vi "toml_read_variant.vi"(7 "section":string[](array[string]), 8 "error in (no error)":errorcluster, 9 "default":variant, 10 "key":string[](array[string]), 11 "path in":path) -> (0 "error out":errorcluster, 1 "value":variant, 2 "exists?":bool, 3 "path out":path)   [LabVIEW 2017]
uses:
  <vilib>/Utility/Data Type/NI_Data Type.lvlib
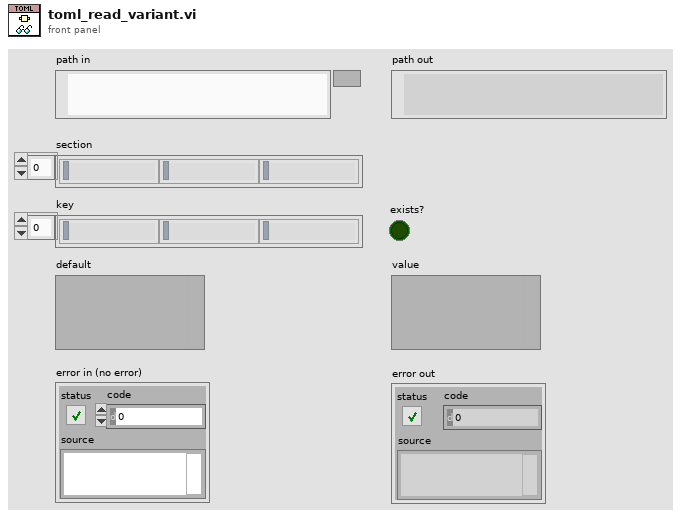
[diagram p1: front panel]
types:
  T1 = typedef "NI_Data Type.lvlib/Data Type.ctl" = enum8{"Invalid Type", "Void", "I8", "I16", "I32", "I64", "U8", "U16", "U32", "U64", "Single Float", "Double Float", "Extended Float", "Single Complex", "Double Complex", "Extended Complex", "Enum U8", "Enum U16", "Enum U32", "Enum U64", "Single Float With Unit", "Double Float With Unit", "Extended Float With Unit", "Single Complex with Unit", "Double Complex with Unit", "Extended Complex with Unit", "Boolean", "String", "Path", "Picture", "Tag", "Array", "Cluster", "Variant", "LV Variant", "Waveform", "Timestamp", "Digital Waveform", "Digital Data", "ExpressData", "Refnum", "External Data", "VI", "Poly VI", "LabVIEW Class Instance", "Fixed Point"}
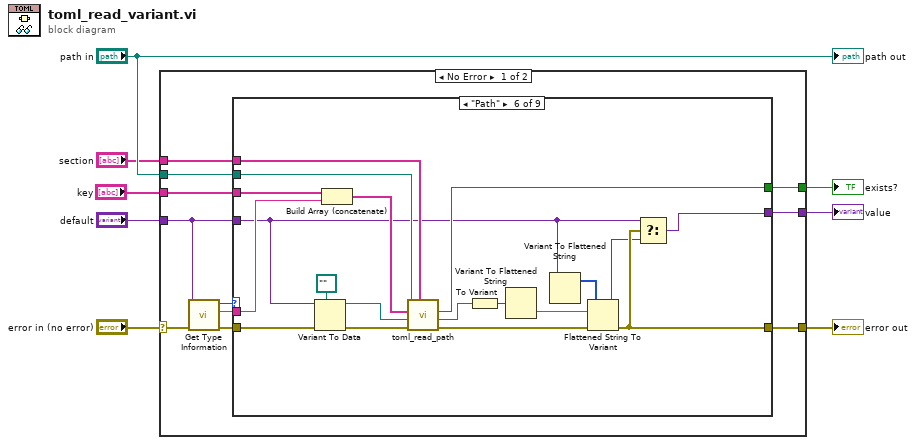
[diagram p0: block diagram]
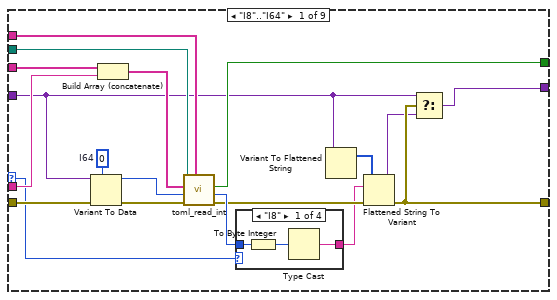
[diagram p2: hidden frame]
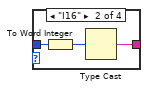
[diagram p3: hidden frame]
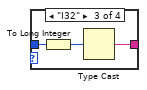
[diagram p4: hidden frame]
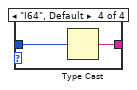
[diagram p5: hidden frame]
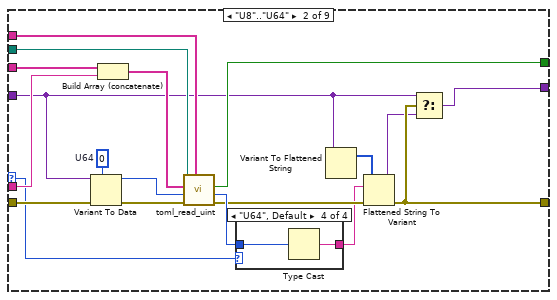
[diagram p6: hidden frame]
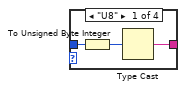
[diagram p7: hidden frame]
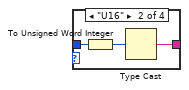
[diagram p8: hidden frame]
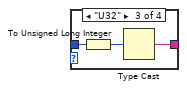
[diagram p9: hidden frame]
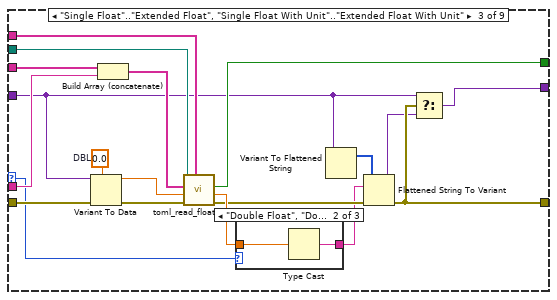
[diagram p10: hidden frame]
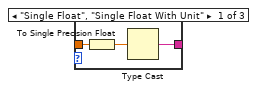
[diagram p11: hidden frame]
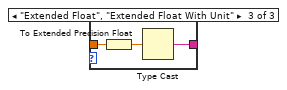
[diagram p12: hidden frame]
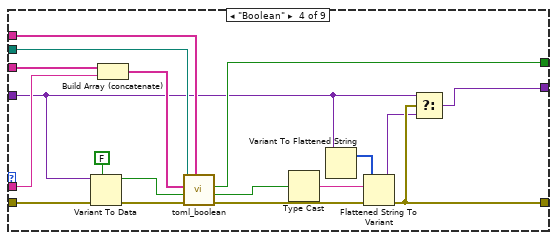
[diagram p13: hidden frame]
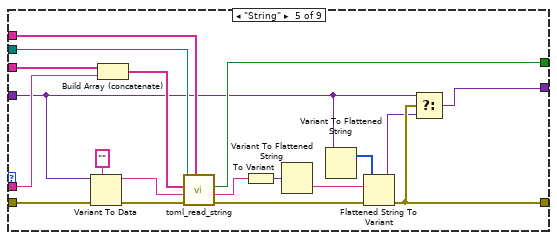
[diagram p14: hidden frame]
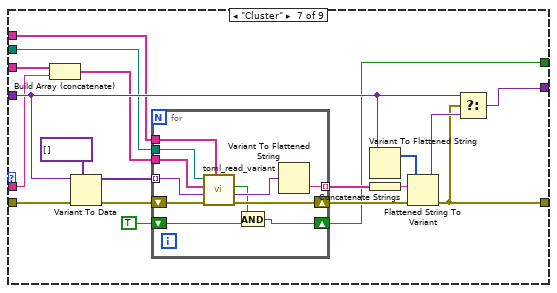
[diagram p15: hidden frame]
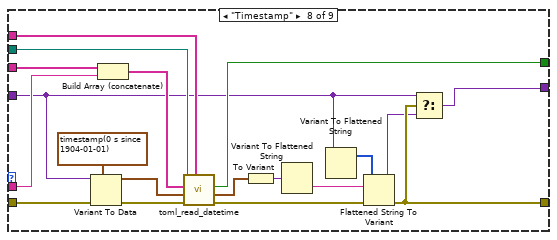
[diagram p16: hidden frame]
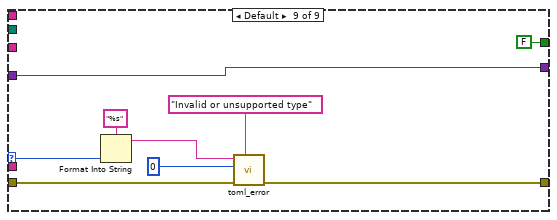
[diagram p17: hidden frame]
diagram:
  n1 = case shown="No Error" "error in (no error)" {
    selector: "error in (no error)" -> [w18 w222]
    tunnel: [w19 w222] -> w8
    tunnel: "default" -> [w16 w221]
    tunnel: [w14 w221] -> w5
    tunnel: "path in" -> [w13 _]
    tunnel: "section" -> [w11 _]
    tunnel: "key" -> [w10 _]
    tunnel: [w9 _] -> w1
    frame No Error {
      n2 = call <vilib>:"Get Type Information.vi"("error in (no error)"=w18, "Variant"=w16) -> ("error out"=w17:errorcluster, "Name"=w12:string, "Type"=w15:T1)  [unwired: 5 in, 2 out]
      n3 = case shown="\"Path\"" w15 {
        selector: w15 -> [w25 w55 w85 _ _ _ _ _ w216]
        tunnel: [w23 w53 w83 w110 w131 w150 w175 w199 w219] -> w19
        tunnel: w17 -> [w38 w68 w98 w124 w143 w162 w181 w211 w220]
        tunnel: w16 -> [w22 w52 w82 w109 w130 w149 w173 w198 w213]
        tunnel: [w20 w50 w80 w107 w128 w147 w174 w196 w213] -> w14
        tunnel: w13 -> [w37 w67 w97 w123 w142 w161 w169 w210 _]
        tunnel: w12 -> [w34 w64 w94 w120 w139 w158 w171 w207 _]
        tunnel: w11 -> [w36 w66 w96 w122 w141 w160 w168 w209 _]
        tunnel: w10 -> [w35 w65 w95 w121 w140 w159 w172 w208 _]
        tunnel: [w29 w59 w89 w115 w134 w153 w163 w202 FALSE ("exists?")] -> w9
        frame "I8".."I64" {
          w31 = i64 0  # I64
          n4 = Variant To Data(error in=w38, type=w31, Variant=w22) -> (data=w30:i64, error out=w32:errorcluster)
          n5 = Build Array (concatenate)(w35, w34) -> (w33:string[])
          n6 = call "toml_read_int.vi"("section"=w36, "error in (no error)"=w32, "default"=w30, "key"=w33, "path in"=w37) -> ("error out"=w27:errorcluster, "value"=w28:i64, "exists?"=w29:bool)  [unwired: 2 in, 2 out]
          n7 = case shown="\"I8\"" w25 {
            tunnel: [w39 w42 w45 w49] -> w24
            tunnel: w28 -> [w41 w44 w47 w48]
            frame "I8" {
              n8 = To Byte Integer(number=w41) -> (8bit integer=w40:i8)
              n9 = Type Cast(x=w40) -> (*(type *) &x=w39:string)  [unwired: 1 in]
            }
            frame "I16" {
              n10 = To Word Integer(number=w44) -> (16bit integer=w43:i16)
              n11 = Type Cast(x=w43) -> (*(type *) &x=w42:string)  [unwired: 1 in]
            }
            frame "I32" {
              n12 = To Long Integer(number=w47) -> (32bit integer=w46:i32)
              n13 = Type Cast(x=w46) -> (*(type *) &x=w45:string)  [unwired: 1 in]
            }
            frame "I64", Default {
              n14 = Type Cast(x=w48) -> (*(type *) &x=w49:string)  [unwired: 1 in]
            }
          }
          n15 = Variant To Flattened String(Variant=w22) -> (1:w26:i16[])  [unwired: 1 out]
          n16 = Flattened String To Variant(4:w27, 6:w24, 7:w26) -> (0:w23:errorcluster, 3:w21:variant)
          n17 = Select(t=w22, s=w23, f=w21) -> (s? t:f=w20:variant)
        }
        frame "U8".."U64" {
          w61 = u64 0  # U64
          n18 = Variant To Data(error in=w68, type=w61, Variant=w52) -> (data=w60:u64, error out=w62:errorcluster)
          n19 = Build Array (concatenate)(w65, w64) -> (w63:string[])
          n20 = call "toml_read_uint.vi"("section"=w66, "error in (no error)"=w62, "default"=w60, "key"=w63, "path in"=w67) -> ("error out"=w57:errorcluster, "value"=w58:u64, "exists?"=w59:bool)  [unwired: 3 in, 1 out]
          n21 = case shown="\"U64\", Default" w55 {
            tunnel: [w69 w72 w75 w79] -> w54
            tunnel: w58 -> [w71 w74 w77 w78]
            frame "U8" {
              n22 = To Unsigned Byte Integer(number=w71) -> (unsigned 8bit integer=w70:u8)
              n23 = Type Cast(x=w70) -> (*(type *) &x=w69:string)  [unwired: 1 in]
            }
            frame "U16" {
              n24 = To Unsigned Word Integer(number=w74) -> (unsigned 16bit integer=w73:u16)
              n25 = Type Cast(x=w73) -> (*(type *) &x=w72:string)  [unwired: 1 in]
            }
            frame "U32" {
              n26 = To Unsigned Long Integer(number=w77) -> (unsigned 32bit integer=w76:u32)
              n27 = Type Cast(x=w76) -> (*(type *) &x=w75:string)  [unwired: 1 in]
            }
            frame "U64", Default {
              n28 = Type Cast(x=w78) -> (*(type *) &x=w79:string)  [unwired: 1 in]
            }
          }
          n29 = Variant To Flattened String(Variant=w52) -> (1:w56:i16[])  [unwired: 1 out]
          n30 = Flattened String To Variant(4:w57, 6:w54, 7:w56) -> (0:w53:errorcluster, 3:w51:variant)
          n31 = Select(t=w52, s=w53, f=w51) -> (s? t:f=w50:variant)
        }
        frame "Single Float".."Extended Float", "Single Float With Unit".."Extended Float With Unit" {
          w91 = 0.0  # DBL
          n32 = Variant To Data(error in=w98, type=w91, Variant=w82) -> (data=w90:dbl, error out=w92:errorcluster)
          n33 = Build Array (concatenate)(w95, w94) -> (w93:string[])
          n34 = call "toml_read_float.vi"("section"=w96, "error in (no error)"=w92, "default"=w90, "key"=w93, "path in"=w97) -> ("error out"=w87:errorcluster, "value"=w88:dbl, "exists?"=w89:bool)  [unwired: 3 in, 1 out]
          n35 = case shown="\"Double Float\", \"Double Float With Unit\", Default" w85 {
            tunnel: [w99 w103 w106] -> w84
            tunnel: w88 -> [w101 w102 w105]
            frame "Single Float", "Single Float With Unit" {
              n36 = To Single Precision Float(number=w101) -> (single precision float=w100:sgl)
              n37 = Type Cast(x=w100) -> (*(type *) &x=w99:string)  [unwired: 1 in]
            }
            frame "Double Float", "Double Float With Unit", Default {
              n38 = Type Cast(x=w102) -> (*(type *) &x=w103:string)  [unwired: 1 in]
            }
            frame "Extended Float", "Extended Float With Unit" {
              n39 = To Extended Precision Float(1:w105) -> (0:w104:ext)
              n40 = Type Cast(x=w104) -> (*(type *) &x=w106:string)  [unwired: 1 in]
            }
          }
          n41 = Variant To Flattened String(Variant=w82) -> (1:w86:i16[])  [unwired: 1 out]
          n42 = Flattened String To Variant(4:w87, 6:w84, 7:w86) -> (0:w83:errorcluster, 3:w81:variant)
          n43 = Select(t=w82, s=w83, f=w81) -> (s? t:f=w80:variant)
        }
        frame "Boolean" {
          n44 = Variant To Data(error in=w124, type=FALSE, Variant=w109) -> (data=w116:bool, error out=w118:errorcluster)
          n45 = Build Array (concatenate)(w121, w120) -> (w119:string[])
          n46 = call "toml_boolean.vi"("section"=w122, "error in (no error)"=w118, "default"=w116, "key"=w119, "path in"=w123) -> ("error out"=w113:errorcluster, "value"=w114:bool, "exists?"=w115:bool)  [unwired: 3 in, 1 out]
          n47 = Type Cast(x=w114) -> (*(type *) &x=w111:string)  [unwired: 1 in]
          n48 = Variant To Flattened String(Variant=w109) -> (1:w112:i16[])  [unwired: 1 out]
          n49 = Flattened String To Variant(4:w113, 6:w111, 7:w112) -> (0:w110:errorcluster, 3:w108:variant)
          n50 = Select(t=w109, s=w110, f=w108) -> (s? t:f=w107:variant)
        }
        frame "String" {
          n51 = Variant To Data(error in=w143, type="", Variant=w130) -> (data=w135:string, error out=w137:errorcluster)
          n52 = Build Array (concatenate)(w140, w139) -> (w138:string[])
          n53 = call "toml_read_string.vi"("section"=w141, "error in (no error)"=w137, "default"=w135, "key"=w138, "path in"=w142) -> ("error out"=w133:errorcluster, "value"=w127:string, "exists?"=w134:bool)  [unwired: 3 in, 1 out]
          n54 = To Variant(anything=w127) -> (Variant=w125:variant)
          n55 = Variant To Flattened String(Variant=w125) -> (data string=w126:string)  [unwired: 1 out]
          n56 = Variant To Flattened String(Variant=w130) -> (1:w132:i16[])  [unwired: 1 out]
          n57 = Flattened String To Variant(4:w133, 6:w126, 7:w132) -> (0:w131:errorcluster, 3:w129:variant)
          n58 = Select(t=w130, s=w131, f=w129) -> (s? t:f=w128:variant)
        }
        frame "Path" {
          n59 = Variant To Data(error in=w162, type=path "", Variant=w149) -> (data=w154:path, error out=w156:errorcluster)
          n60 = Build Array (concatenate)(w159, w158) -> (w157:string[])
          n61 = call "toml_read_path.vi"("section"=w160, "error in (no error)"=w156, "default"=w154, "key"=w157, "path in"=w161) -> ("error out"=w152:errorcluster, "value"=w146:path, "exists?"=w153:bool)  [unwired: 3 in, 1 out]
          n62 = To Variant(anything=w146) -> (Variant=w144:variant)
          n63 = Variant To Flattened String(Variant=w144) -> (data string=w145:string)  [unwired: 1 out]
          n64 = Variant To Flattened String(Variant=w149) -> (1:w151:i16[])  [unwired: 1 out]
          n65 = Flattened String To Variant(4:w152, 6:w145, 7:w151) -> (0:w150:errorcluster, 3:w148:variant)
          n66 = Select(t=w149, s=w150, f=w148) -> (s? t:f=w147:variant)
        }
        frame "Cluster" {
          n67 = Build Array (concatenate)(w172, w171) -> (w170:string[])
          n68 = Variant To Data(error in=w181, type=variant[] [], Variant=w173) -> (data=w167:variant[], error out=w179:errorcluster)
          n69 = for {
            shift-right: [w191] -> w176
            shift-left: w179 -> [w192]
            tunnel: w170 -> [w190]
            tunnel: w169 -> [w189]
            tunnel: w168 -> [w188]
            tunnel: w167 -> [w187] mode=indexing
            tunnel: [w185] -> w166 mode=indexing
            shift-right: [w182] -> w163
            shift-left: TRUE -> [w183]
            n70 = call "toml_read_variant.vi"("section"=w188, "error in (no error)"=w192, "default"=w187, "key"=w190, "path in"=w189) -> ("error out"=w191:errorcluster, "value"=w186:variant, "exists?"=w184:bool)  [unwired: 3 in, 1 out]
            n71 = And(x=w184, y=w183) -> (x .and. y?=w182:bool)
            n72 = Variant To Flattened String(Variant=w186) -> (data string=w185:string)  [unwired: 1 out]
          }
          n73 = Variant To Flattened String(Variant=w173) -> (1:w178:i16[])  [unwired: 1 out]
          n74 = Concatenate Strings(w166) -> (w165:string)
          n75 = Flattened String To Variant(4:w176, 6:w165, 7:w178) -> (0:w175:errorcluster, 3:w177:variant)
          n76 = Select(t=w173, s=w175, f=w177) -> (s? t:f=w174:variant)
        }
        frame "Timestamp" {
          n77 = Variant To Data(error in=w211, type=timestamp(0 s since 1904-01-01), Variant=w198) -> (data=w203:timestamp, error out=w205:errorcluster)
          n78 = Build Array (concatenate)(w208, w207) -> (w206:string[])
          n79 = call "toml_read_datetime.vi"("section"=w209, "error in (no error)"=w205, "default"=w203, "key"=w206, "path in"=w210) -> ("error out"=w201:errorcluster, "value"=w195:timestamp, "exists?"=w202:bool)  [unwired: 3 in, 1 out]
          n80 = To Variant(anything=w195) -> (Variant=w193:variant)
          n81 = Variant To Flattened String(Variant=w193) -> (data string=w194:string)  [unwired: 1 out]
          n82 = Variant To Flattened String(Variant=w198) -> (1:w200:i16[])  [unwired: 1 out]
          n83 = Flattened String To Variant(4:w201, 6:w194, 7:w200) -> (0:w199:errorcluster, 3:w197:variant)
          n84 = Select(t=w198, s=w199, f=w197) -> (s? t:f=w196:variant)
        }
        frame Default {
          n85 = Format Into String(format string="%s", w216) -> (resulting string=w214:string)  [unwired: 2 in, 1 out]
          n86 = call "toml_error.vi"("message"="Invalid or unsupported type", "error in (no error)"=w220, "offset (0)"=0, "toml"=w214) -> ("error out"=w219:errorcluster)  [unwired: 7 in]
        }
      }
    }
    frame Error {
    }
  }
  "error out" <- w8
  "value" <- w5
  "exists?" <- w1
  "path out" <- "path in"
